vi "Read HDF5.vi"(8 "error in (no error)":errorcluster, 10 "path":path, 11 "LVtoITX in":refnum<class "LVtoITX.lvclass">) -> (0 "error out":errorcluster, 1 "Wavenames":string[](array[string]), 2 "Data":dbl[][](array[numeric]), 3 "LVtoITX out":refnum<class "LVtoITX.lvclass">, 4 "Comments":string, 6 "Igor Commands":string)   [LabVIEW 2016, in "LVtoITX.lvclass"]
uses:
  LVtoITX.lvclass
  <vilib>/addons/h5labview2/file/H5Fmode.ctl
  LVtoITX.lvclass/LVtoITX.ctl
  <vilib>/addons/h5labview2/base/lib_path.vi
  <vilib>/addons/h5labview2/base/H5Equery.vi
  <vilib>/addons/h5labview2/dataset/H5Dread.llb/H5Dread.xnode
  <vilib>/addons/h5labview2/file/H5F.lvlib
  <vilib>/addons/h5labview2/group/H5G.lvlib
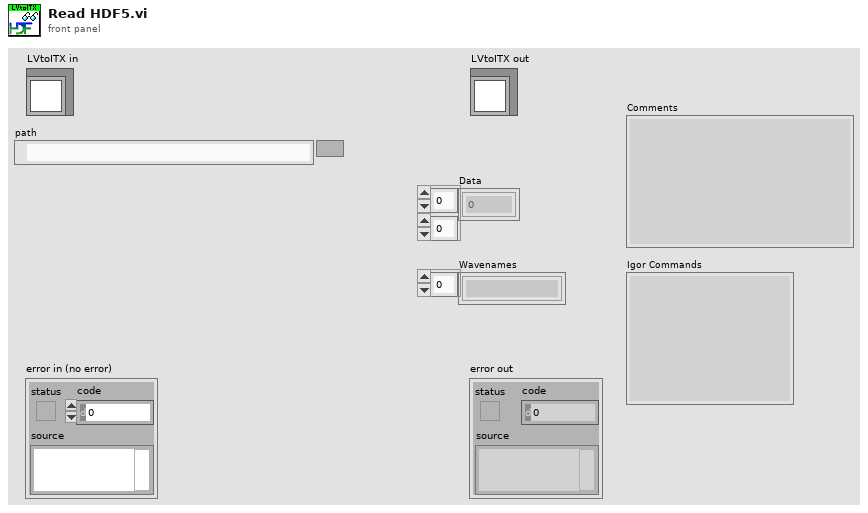
[diagram p1: front panel]
types:
  T1 = typedef "H5F.lvlib/H5Fmode.ctl" = enum16{"read-only", "read-write", "overwrite", "create new", "open or create"}
  T2 = typedef "hid_t.ctl" = i32
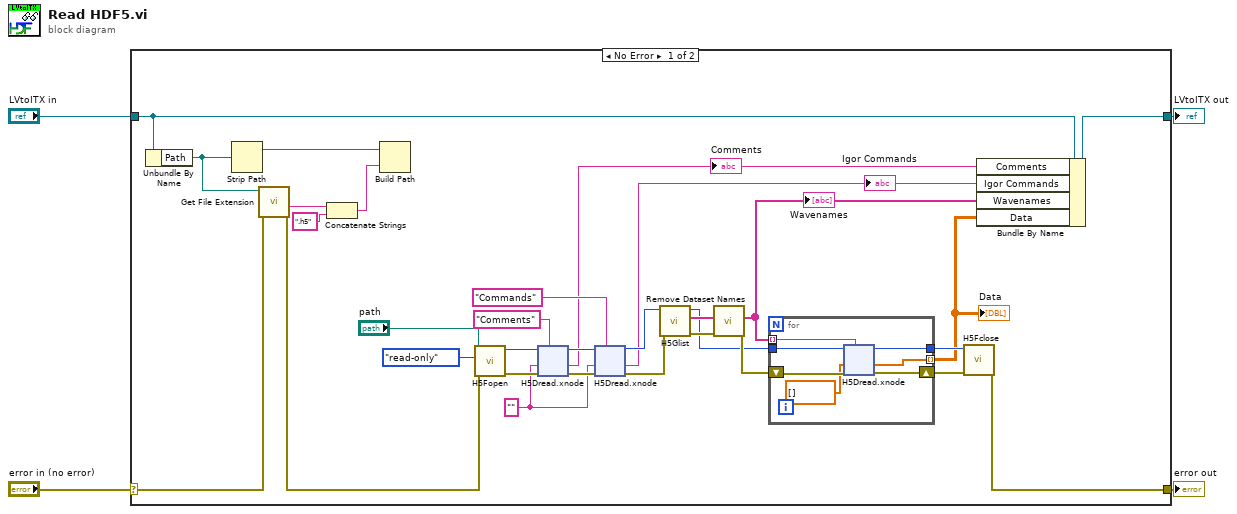
[diagram p0: block diagram]
diagram:
  n1 = case shown="No Error" "error in (no error)" {
    selector: "error in (no error)" -> [w19 w88]
    tunnel: [w24 w88] -> w1
    tunnel: [w20 w89] -> w2
    tunnel: "LVtoITX in" -> [w21 w89]
    frame No Error {
      w5 = "" ("attrib name")
      n2 = Unbundle By Name(w21) -> ("Path"=w23:path)
      n3 = Strip Path(path=w23) -> (stripped path=w32:path)  [unwired: 1 out]
      n4 = call <vilib>:"Get File Extension.vi"("error in (no error)"=w19, "file"=w23) -> ("error out"=w30:errorcluster, "filename without extension"=w34:string)  [unwired: 5 in, 3 out]
      n5 = Concatenate Strings(w34, ".h5" ("string")) -> (w31:string)
      n6 = Build Path(base path=w32, name or relative path=w31) -> ()  [unwired: 1 out]
      n7 = call <vilib>:"H5Fopen.vi"("error in (no error)"=w30, "mode (read-only)"=H5Fmode."read-only" ("mode"), "path"="path") -> ("error out"=w29:errorcluster, "ref out"=w22:T2)  [unwired: 7 in]
      n8 = xnode "H5Dread.xnode"("dataset name (this)"="Comments" ("attrib name"), "error in (no error)"=w29, "default"=w5, "ref in"=w22) -> ("error out"=w27:errorcluster, "data"=w16:string, "ref out"=w26:i32)  [unwired: 2 in, 1 out]
      "Comments" <- w16
      n9 = xnode "H5Dread.xnode"("dataset name (this)"="Commands" ("attrib name"), "error in (no error)"=w27, "default"=w5, "ref in"=w26) -> ("error out"=w8:errorcluster, "data"=w17:string, "ref out"=w18:i32)  [unwired: 2 in, 1 out]
      "Igor Commands" <- w17
      n10 = call <vilib>:"H5Glist.vi"("error in (no error)"=w8, "ref in"=w18) -> ("error out"=w11:errorcluster, "names"=w12:string[], "ref out"=w9:T2)  [unwired: 6 in, 1 out]
      n11 = call "Remove Dataset Names.vi"("error in (no error)"=w11, "Dataset Names"=w12) -> ("error out"=w10:errorcluster, "Name less Commands and Comments"=w6:string[])  [unwired: 8 in]
      "Wavenames" <- w6
      n12 = for {
        shift-right: [w42] -> w14
        shift-left: w10 -> [w41]
        tunnel: w9 -> [w40]
        tunnel: [w39] -> w13
        tunnel: w6 -> [w37] mode=indexing
        tunnel: [w36] -> w7 mode=indexing
        n13 = xnode "H5Dread.xnode"("dataset name (this)"=w37, "error in (no error)"=w41, "default"=dbl[] [] ("array type (2D Dbl)"), "ref in"=w40) -> ("error out"=w42:errorcluster, "data"=w36:dbl[], "ref out"=w39:i32)  [unwired: 2 in, 1 out]
      }
      "Data" <- w7
      n14 = call <vilib>:"H5Fclose.vi"("error in (no error)"=w14, "ref"=w13) -> ("error out"=w24:errorcluster)  [unwired: 9 in]
      n15 = Bundle By Name(cluster=w21, "Comments"=w16, "Igor Commands"=w17, "Wavenames"=w6, "Data"=w7) -> (w20:refnum<class "LVtoITX.lvclass">)
    }
    frame Error {
    }
  }
  "error out" <- w1
  "LVtoITX out" <- w2
